vi "GetStepTreePosition.vi"(8 "error in (no error)":errorcluster, 11 "Node Reference in":refnum<data-value>) -> (0 "error out":errorcluster, 2 "TreeIndex":i32)   [LabVIEW 2015, in "StepNode.lvclass"]
uses:
  StepNode.lvclass
  <vilib>/NI/Configuration Framework/Node/NISE_CEF_Node.lvclass/NISE_CEF_Node.ctl
  <vilib>/NI/Configuration Framework/Node/ReadParent.vi
  <vilib>/NI/Configuration Framework/Node/ReadChildren.vi
  <vilib>/NI/Configuration Framework/Node/NISE_CEF_Node.lvclass
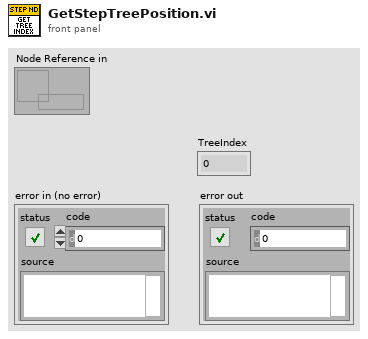
[diagram p1: front panel]
types:
  T1 = typedef "NISE_CEF_Node.lvclass/NodeRef.ctl" = refnum<data-value>
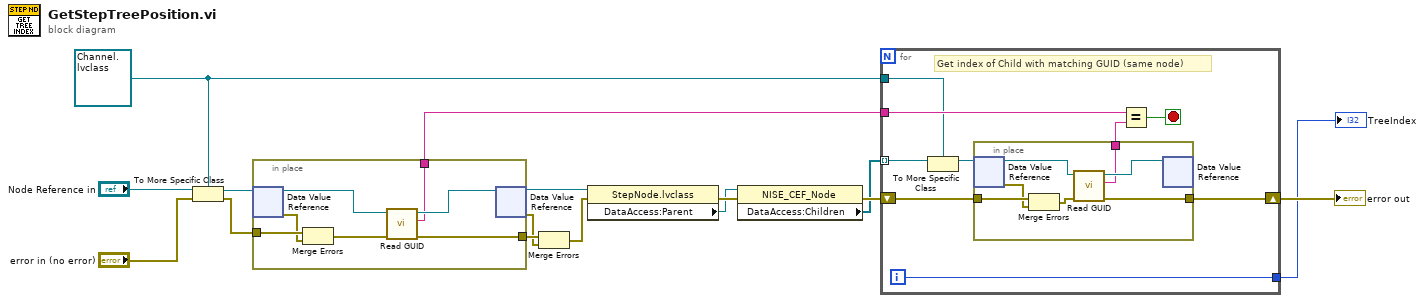
[diagram p0: block diagram]
diagram:
  w1 = refnum<data-value> refnum ("data value reference")
  n1 = To More Specific Class(target class=w1, reference="Node Reference in", error in="error in (no error)") -> (specific class reference=w8:refnum<data-value>, error out=w7:errorcluster)
  n2 = in-place {
    in-place-border: w7 -> [w23]
    in-place-border: [w20] -> w6
    in-place-border: [w17] -> w2
    n3 = in-place-dvr #1(w8) -> (w19:refnum<class "StepNode.lvclass">, w22:errorcluster)
    n4 = Merge Errors(w23, w22) -> (w21:errorcluster)
    n5 = call-dynamic "Read GUID.vi"("error in (no error)"=w21, "StepNode in"=w19) -> ("error out"=w20:errorcluster, "GUID"=w17:string, "StepNode out"=w18:refnum<class "StepNode.lvclass">)  [unwired: 7 in]
    n6 = in-place-dvr #1(w18) -> (w3:refnum<data-value>, w5:errorcluster)
  }
  n7 = Merge Errors(w6, w5) -> (w4:errorcluster)
  n8 = property on="Property Node" class="StepNode.lvclass"(reference=w3, error in=w4) -> (error out=w16:errorcluster, "DataAccess:Parent"=w13:T1)  [unwired: 1 out]
  n9 = property class="NISE_CEF_Node"(reference=w13, error in=w16) -> (error out=w14:errorcluster, "DataAccess:Children"=w11:T1[])  [unwired: 1 out]
  n10 = for {
    shift-right: [w31] -> w12
    shift-left: w14 -> [w32]
    tunnel: w11 -> [w30] mode=indexing
    tunnel: [w26] -> w10
    tunnel: w2 -> [w25]
    tunnel: w1 -> [w24]
    i -> [w26]
    stop <- w27 stop-if-true
    # "Get index of Child with matching GUID (same node)"
    n11 = To More Specific Class(target class=w24, reference=w30) -> (specific class reference=w29:refnum<data-value>)  [unwired: 1 in, 1 out]
    n12 = in-place {
      in-place-border: w32 -> [w39]
      in-place-border: [w38] -> w31
      in-place-border: [w34] -> w28
      n13 = in-place-dvr #2(w29) -> (w33:refnum<class "StepNode.lvclass">, w35:errorcluster)
      n14 = Merge Errors(w39, w35) -> (w36:errorcluster)
      n15 = call-dynamic "Read GUID.vi"("error in (no error)"=w36, "StepNode in"=w33) -> ("error out"=w38:errorcluster, "GUID"=w34:string, "StepNode out"=w37:refnum<class "StepNode.lvclass">)  [unwired: 7 in]
      n16 = in-place-dvr #2(w37) -> ()  [unwired: 2 out]
    }
    n17 = Equal?(x=w25, y=w28) -> (x = y?=w27:bool)
  }
  "error out" <- w12
  "TreeIndex" <- w10
